vi "Read Read Directory.vi"(8 "error in (no error)":errorcluster, 11 "shared memory configuration in":refnum<class "Shared Memory Configuration.lvclass">) -> (0 "error out":errorcluster, 2 "read directory":path, 3 "shared memory configuration out":refnum<class "Shared Memory Configuration.lvclass">)   [LabVIEW 2013]
uses:
  shared memory configuration.lvclass
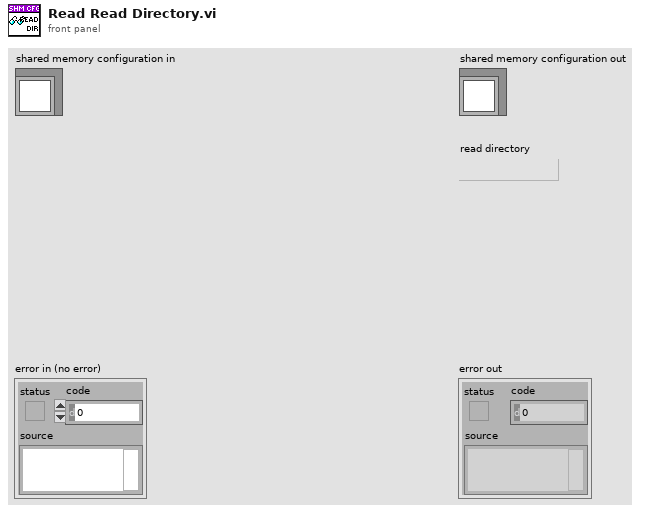
[diagram p1: front panel]
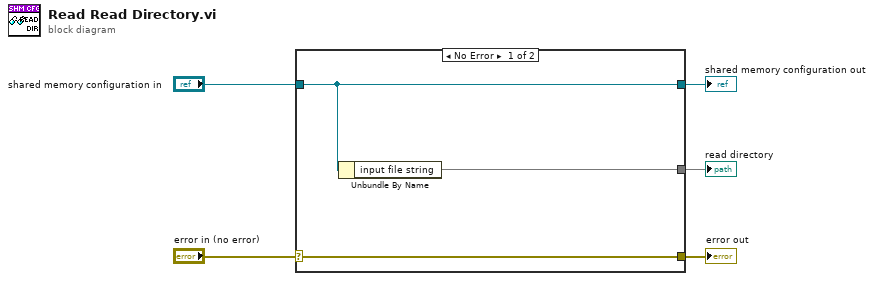
[diagram p0: block diagram]
diagram:
  n1 = case shown="No Error" "error in (no error)" {
    selector: "error in (no error)" -> [w8 w9]
    tunnel: [w8 w9] -> w4
    tunnel: [w7 w10] -> w2
    tunnel: "shared memory configuration in" -> [w7 w10]
    tunnel: [w6 _] -> w1
    frame No Error {
      n2 = Unbundle By Name(w7) -> ("input file string"=w6)
    }
    frame Error {
    }
  }
  "error out" <- w4
  "shared memory configuration out" <- w2
  "read directory" <- w1
